vi "仪器初始化.vi"(8 "错误输入（无错误）":errorcluster, 11 "仪器地址":T1) -> (0 "error out":errorcluster, 3 "仪器实例 out":T2)   [LabVIEW 2020]
uses:
  <instrlib>/Keithley 27XX/Keithley 27XX.lvlib
  S7_1200 control/S7_1200 control.lvlib
  <instrlib>/IT6300/IT6300.lvlib
  <instrlib>/Keithley 24XX/Keithley 24XX.lvlib
  F:/F020/S7_1200 control/HslCommunication.dll
  S7_1200 control/HslCommunication.dll
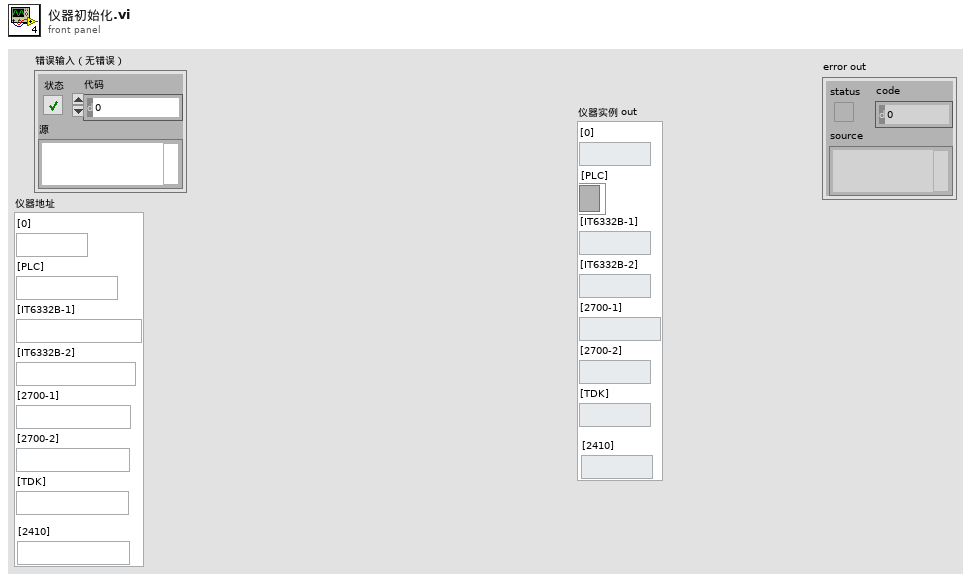
[diagram p1: front panel]
types:
  T1 = typedef "仪器地址输入.ctl" = cluster{"[0]":string, "[PLC]":string, "[IT6332B-1]":string, "[IT6332B-2]":string, "[2700-1]":string, "[2700-2]":string, "[TDK]":string, "[2410]":string}
  T2 = typedef "仪器实例.ctl" = cluster{"[0]":string, "[PLC]":refnum<k24>, "[IT6332B-1]":string, "[IT6332B-2]":string, "[2700-1]":string, "[2700-2]":string, "[TDK]":string, "[2410]":string}
  T3 = cluster{"Channel1":bool, "Channel2":bool, "Channel3":bool}
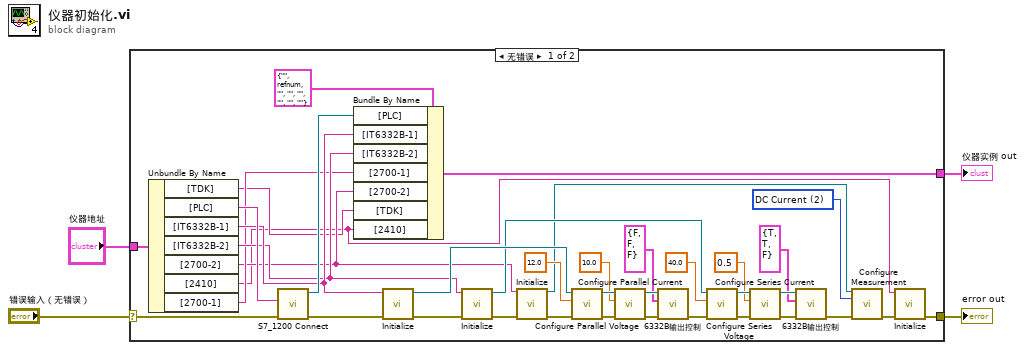
[diagram p0: block diagram]
diagram:
  n1 = case shown="无错误" "错误输入（无错误）" {
    selector: "错误输入（无错误）" -> [w22 w43]
    tunnel: "仪器地址" -> [w42 _]
    tunnel: [w20 w43] -> w4
    tunnel: [w41 _] -> w3
    frame No Error {
      w40 = u16 2 items=["DC Voltage", "AC Voltage", "DC Current", "AC Current", "Resistance", "Four-Wire Resistance", "Temperature", "Frequency", "Period", "Continuity"] ("Function (0: DC Voltage)")
      n2 = Unbundle By Name(w42) -> ("[TDK]"=w6:string, "[PLC]"=w39:string, "[IT6332B-1]"=w10:string, "[IT6332B-2]"=w9:string, "[2700-2]"=w7:string, "[2410]"=w5:string, "[2700-1]"=w8:string)
      n3 = call "S7_1200 Connect.vi"("错误输入（无错误）"=w22, "ipAddress"=w39) -> ("错误输出"=w38:errorcluster, "引用输出"=w23:refnum<k24>)  [unwired: 4 in]
      n4 = Bundle By Name(cluster=T2 {"[0]"="", "[PLC]"=refnum, "[IT6332B-1]"="", "[IT6332B-2]"="", "[2700-1]"="", "[2700-2]"="", "[TDK]"="", "[2410]"=""} ("仪器实例 out"), "[PLC]"=w23, "[IT6332B-1]"=w10, "[IT6332B-2]"=w9, "[2700-1]"=w8, "[2700-2]"=w7, "[TDK]"=w6, "[2410]"=w5) -> (w41:T2)
      n5 = call <instrlib>:"Initialize.vi"("error in (no error)"=w38, "VISA resource name"=w10) -> ("error out"=w37:errorcluster, "VISA resource name out"=w27:refnum<visa-resource-name>)  [unwired: 8 in]
      n6 = call <instrlib>:"Initialize.vi"("error in (no error)"=w37, "VISA resource name"=w9) -> ("error out"=w36:errorcluster, "VISA resource name out"=w26:refnum<visa-resource-name>)  [unwired: 8 in]
      n7 = call <instrlib>:"Initialize.vi"("VISA resource name"=w7, "error in (no error)"=w36) -> ("VISA resource name out"=w24:refnum<visa-resource-name>, "error out"=w25:errorcluster)  [unwired: 12 in]
      n8 = call <instrlib>:"Configure Parallel Voltage.vi"("error in (no error)"=w25, "Voltage Level (0.0 V)"=12.0, "VISA resource name"=w27) -> ("error out"=w35:errorcluster, "VISA resource name out"=w34:refnum<visa-resource-name>)  [unwired: 7 in]
      n9 = call <instrlib>:"Configure Parallel Current.vi"("error in (no error)"=w35, "Current Level (0.0 A)"=10.0, "VISA resource name"=w34) -> ("error out"=w16:errorcluster, "VISA resource name out"=w18:refnum<visa-resource-name>)  [unwired: 7 in]
      n10 = call "6332B输出控制.vi"("错误输入"=w16, "Choose Channel"=T3 {"Channel1"=FALSE, "Channel2"=FALSE, "Channel3"=FALSE}, "VISA资源名称"=w18) -> ("错误输出"=w17:errorcluster)  [unwired: 7 in, 1 out]
      n11 = call <instrlib>:"Configure Series Voltage.vi"("error in (no error)"=w17, "Voltage Level (0.0 V)"=40.0, "VISA resource name"=w26) -> ("error out"=w33:errorcluster, "VISA resource name out"=w32:refnum<visa-resource-name>)  [unwired: 7 in]
      n12 = call <instrlib>:"Configure Series Current.vi"("error in (no error)"=w33, "Current Level (0.0 A)"=0.5, "VISA resource name"=w32) -> ("error out"=w14:errorcluster, "VISA resource name out"=w12:refnum<visa-resource-name>)  [unwired: 7 in]
      n13 = call "6332B输出控制.vi"("错误输入"=w14, "Choose Channel"=T3 {"Channel1"=TRUE, "Channel2"=TRUE, "Channel3"=FALSE}, "VISA资源名称"=w12) -> ("错误输出"=w13:errorcluster)  [unwired: 7 in, 1 out]
      n14 = call <instrlib>:"Configure Measurement.vi"("VISA resource name"=w24, "Function (0: DC Voltage)"=w40, "error in (no error)"=w13) -> ("error out"=w21:errorcluster)  [unwired: 11 in, 1 out]
      n15 = call <instrlib>:"Initialize.vi"("error in (no error)"=w21, "VISA resource name"=w5) -> ("error out"=w20:errorcluster)  [unwired: 8 in, 1 out]
    }
    frame Error {
    }
  }
  "error out" <- w4
  "仪器实例 out" <- w3
